vi "Coils.vi"(0 "Handle In":u64[](array[numeric]), 1 "Device ID":u8=1, 2 "Read Start":u16=17, 3 "Read Amount":u16=16, 4 "Write Start":u16=1, 5 "Write Amount":u16=16, 6 "WR Data":u8[](array[numeric]), 7 "Operation":enum16{"Read", "Write", "Read/Write"}(ring), 8 "error in (no error)":errorcluster) -> (18 "error out":errorcluster, 20 "Handle Out":u64[](array[numeric]), 21 "Result":i32, 22 "RD Data":u8[](array[numeric]))   [LabVIEW 2020]
uses:
  windows/snapmb.dll
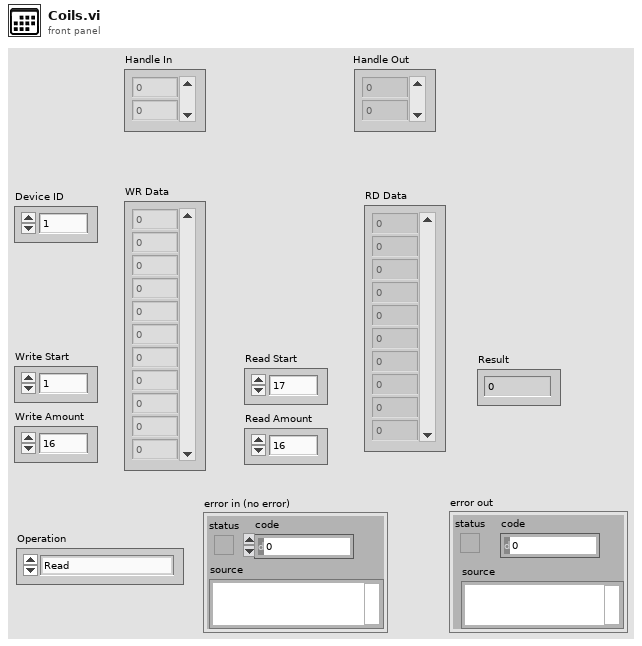
[diagram p1: front panel]
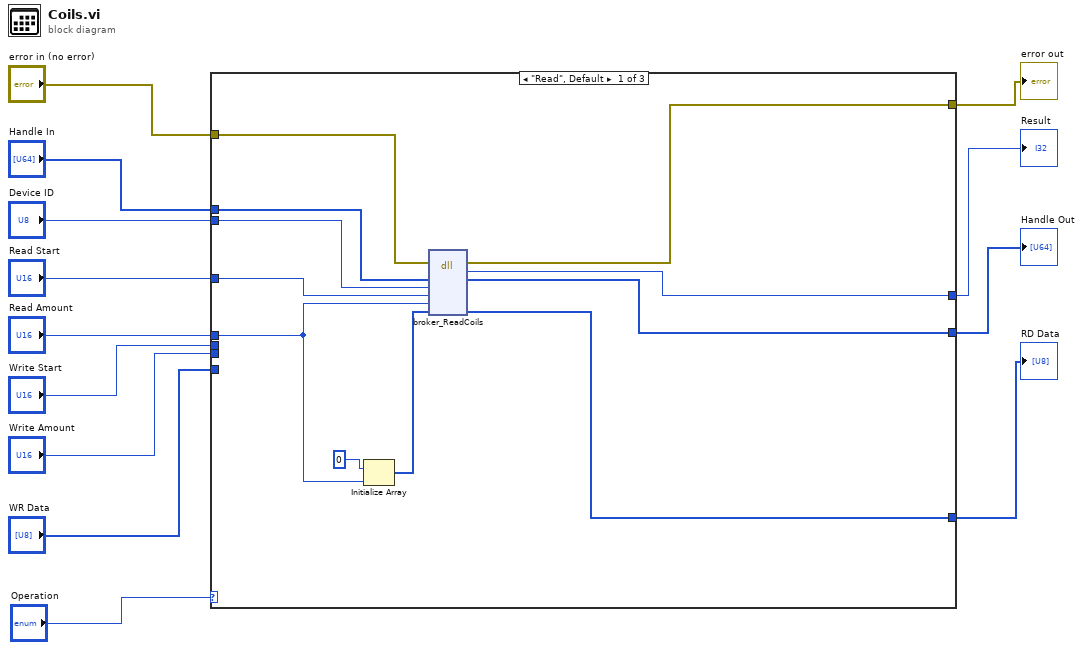
[diagram p0: block diagram]
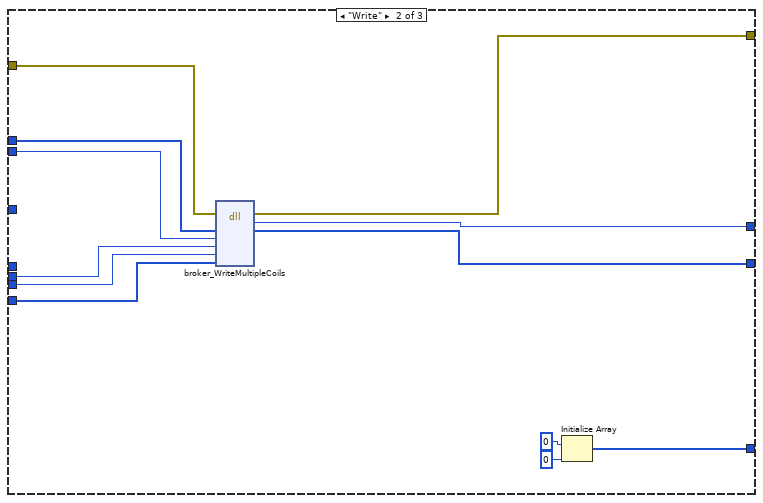
[diagram p2: hidden frame]
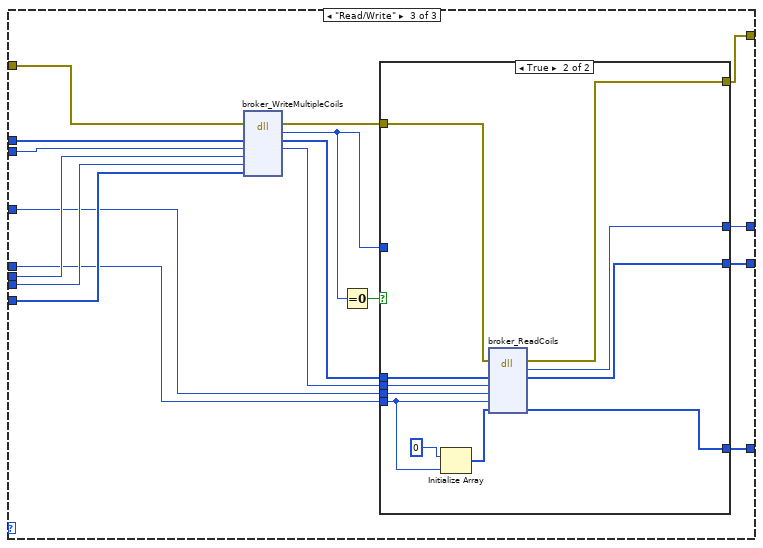
[diagram p3: hidden frame]
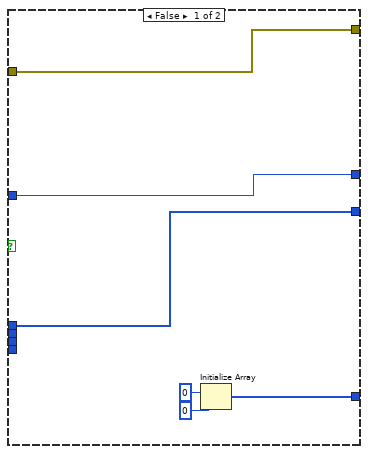
[diagram p4: hidden frame]
diagram:
  n1 = case shown="\"Read\", Default" "Operation" {
    tunnel: "Handle In" -> [w19 w35 w49]
    tunnel: "Device ID" -> [w20 w34 w48]
    tunnel: "Read Start" -> [w21 _ w43]
    tunnel: "Read Amount" -> [w22 _ w42]
    tunnel: "Write Start" -> [_ w33 w53]
    tunnel: "Write Amount" -> [_ w32 w52]
    tunnel: "WR Data" -> [_ w31 w51]
    tunnel: [w18 w30 w47] -> w5
    tunnel: [w15 w29 w44] -> w4
    tunnel: "error in (no error)" -> [w17 w36 w40]
    tunnel: [w16 w28 w39] -> w2
    tunnel: [w14 w25 w37] -> w1
    frame "Read", Default {
      n2 = Initialize Array(u8 0 ("element"), w22) -> (w23:u8[])
      n3 = dll-call lib="D:/SnapMB/LabView/lib/windows/snapmb.dll" fn="broker_ReadCoils"(error in=w17, "Handle"=w19, "DeviceID"=w20, "Start"=w21, "Amount"=w22, "pUsrData"=w23) -> (error out=w16:errorcluster, "Result"=w18:i32, "Handle"=w15:u64[], "pUsrData"=w14:u8[])  [unwired: 5 in, 1 out]
    }
    frame "Write" {
      n4 = dll-call lib="D:/SnapMB/LabView/lib/windows/snapmb.dll" fn="broker_WriteMultipleCoils"(error in=w36, "Handle"=w35, "DeviceID"=w34, "Start"=w33, "Amount"=w32, "pUsrData"=w31) -> (error out=w28:errorcluster, "Result"=w30:i32, "Handle"=w29:u64[])  [unwired: 6 in, 1 out]
      n5 = Initialize Array(u8 0 ("element"), 0 ("dimension size")) -> (w25:u8[])
    }
    frame "Read/Write" {
      n6 = dll-call lib="D:/SnapMB/LabView/lib/windows/snapmb.dll" fn="broker_WriteMultipleCoils"(error in=w40, "Handle"=w49, "DeviceID"=w48, "Start"=w53, "Amount"=w52, "pUsrData"=w51) -> (error out=w38:errorcluster, "Result"=w46:i32, "Handle"=w45:u64[], "DeviceID"=w41:u8)  [unwired: 5 in, 1 out]
      n7 = Equal To 0?(x=w46) -> (x = 0?=w50:bool)
      n8 = case shown="True" w50 {
        tunnel: [w58 w70] -> w47
        tunnel: w46 -> [w58 _]
        tunnel: w45 -> [w59 w69]
        tunnel: [w59 w68] -> w44
        tunnel: w43 -> [_ w65]
        tunnel: w42 -> [_ w63]
        tunnel: w41 -> [_ w64]
        tunnel: [w55 w62] -> w39
        tunnel: w38 -> [w55 w61]
        tunnel: [w54 w60] -> w37
        frame False {
          n9 = Initialize Array(u8 0 ("element"), 0 ("dimension size")) -> (w54:u8[])
        }
        frame True {
          n10 = Initialize Array(u8 0 ("element"), w63) -> (w66:u8[])
          n11 = dll-call lib="D:/SnapMB/LabView/lib/windows/snapmb.dll" fn="broker_ReadCoils"(error in=w61, "Handle"=w69, "DeviceID"=w64, "Start"=w65, "Amount"=w63, "pUsrData"=w66) -> (error out=w62:errorcluster, "Result"=w70:i32, "Handle"=w68:u64[], "pUsrData"=w60:u8[])  [unwired: 5 in, 1 out]
        }
      }
    }
  }
  "Result" <- w5
  "RD Data" <- w1
  "Handle Out" <- w4
  "error out" <- w2
